vi "TagDB Write Data Example.vi"() -> ()   [LabVIEW 2017]
uses:
  TagDB Application Example/DEF-SineSettings.ctl
  9d9cadb0-fa1b-4c2f-b358-df9a280cddfa.vi
  ba25bb52-5bf6-43af-959d-e9a790955eeb.vi
  c988338c-dfcd-45ae-a170-0c12240f6647.vi
  TagDB/_Support/DataAccess/data-Write.vi
  TagDB/_Support/Error/_[error50000]Invalid DB REF.vi
  TagDB/_Support/DataAccess/TagDB Ref to DVR.vi
  TagDB/_Support/DataAccess/_NameCacher.vi
  TagDB/_Support/DataAccess/_datatypeChecker.vi
  <vilib>/Utility/Data Type/Get Type Information.vi
  TagDB/_Support/Error/_Build Error Cluster.vi
  TagDB/TagDB.lvlib
panel:
  out "Write Tag":string[](array[string])
  out "Write Data Recursive":string[](array[string])
  out "Write Data Elements":string[](array[string])
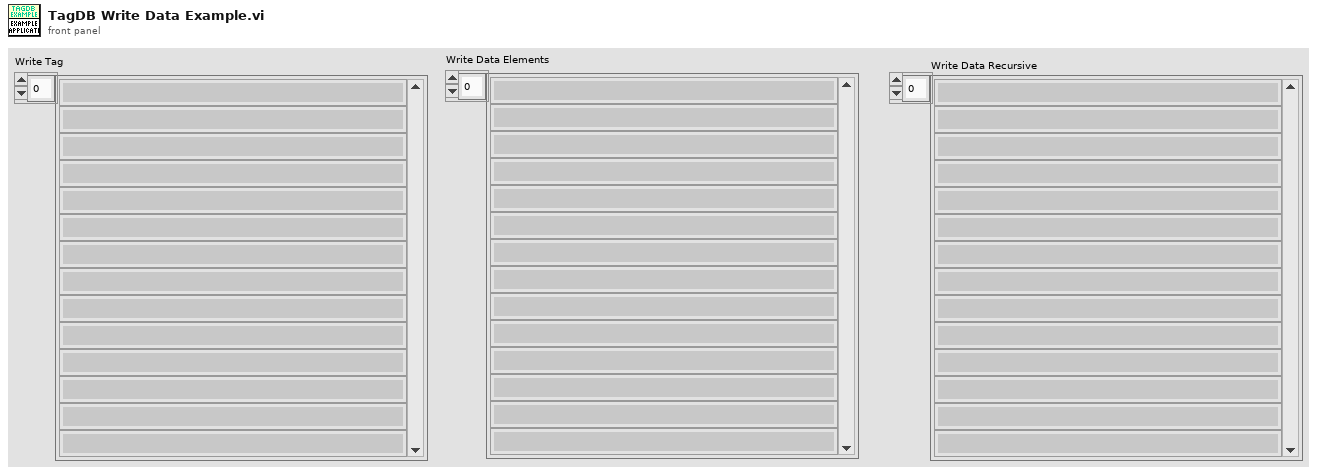
[diagram p1: front panel]
types:
  T1 = typedef "DEF-SineSettings.ctl" = cluster{"frequency":dbl, "amplitude":dbl, "phase":dbl, "sampling info":cluster{"Fs":dbl, "#s":dbl}}
  T2 = typedef "TagDB.lvlib/TagDB.ctl" = refnum<k1>
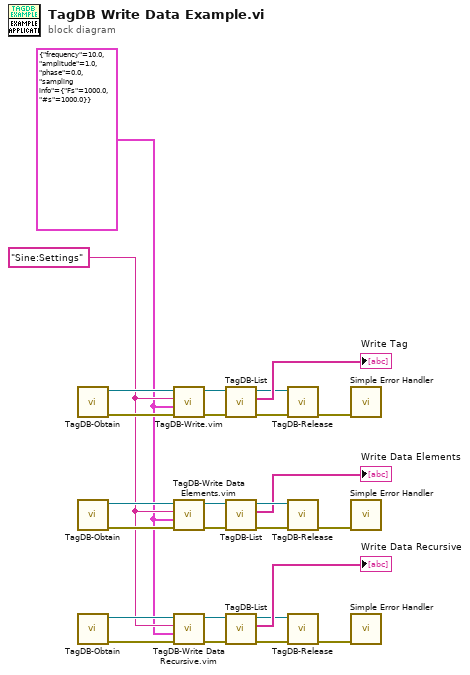
[diagram p0: block diagram]
diagram:
  w2 = "Sine:Settings" ("name")
  w1 = T1 {"frequency"=10.0, "amplitude"=1.0, "phase"=0.0, "sampling info"={"Fs"=1000.0, "#s"=1000.0}} ("Sine Settings")
  n1 = call "TagDB-Obtain.vi"() -> ("error out"=w5:errorcluster, "TagDB"=w4:T2)  [unwired: 5 in, 1 out]
  n2 = call "TagDB-Obtain.vi"() -> ("error out"=w24:errorcluster, "TagDB"=w25:T2)  [unwired: 5 in, 1 out]
  n3 = call "TagDB-Obtain.vi"() -> ("error out"=w13:errorcluster, "TagDB"=w12:T2)  [unwired: 5 in, 1 out]
  n4 = call "TagDB-Write.vim"("error in (no error)"=w5, "Value"=w1, "tag"=w2, "TagDB"=w4) -> ("error out"=w8:errorcluster, "TagDB(dup)"=w6:T2)  [unwired: 5 in, 1 out]
  n5 = call "TagDB-Write Data Elements.vim"("error in (no error)"=w24, "Value"=w1, "root tag"=w2, "TagDB"=w25) -> ("error out"=w21:errorcluster, "TagDB(dup)"=w23:T2)  [unwired: 5 in, 1 out]
  n6 = call "TagDB-Write Data Recursive.vim"("error in (no error)"=w13, "Value"=w1, "root tag"=w2, "TagDB"=w12) -> ("error out"=w16:errorcluster, "TagDB(dup)"=w14:T2)  [unwired: 5 in, 1 out]
  n7 = call "TagDB-List.vi"("error in (no error)"=w8, "TagDB"=w6) -> ("error out"=w9:errorcluster, "names"=→"Write Tag":string[], "TagDB(dup)"=w7:T2)  [unwired: 6 in, 1 out]
  n8 = call "TagDB-List.vi"("error in (no error)"=w21, "TagDB"=w23) -> ("error out"=w20:errorcluster, "names"=→"Write Data Elements":string[], "TagDB(dup)"=w22:T2)  [unwired: 6 in, 1 out]
  n9 = call "TagDB-List.vi"("error in (no error)"=w16, "TagDB"=w14) -> ("error out"=w17:errorcluster, "names"=→"Write Data Recursive":string[], "TagDB(dup)"=w15:T2)  [unwired: 6 in, 1 out]
  n10 = call "TagDB-Release.vi"("error in (no error)"=w9, "TagDB"=w7) -> ("error out"=w3:errorcluster)  [unwired: 9 in]
  n11 = call "TagDB-Release.vi"("error in (no error)"=w20, "TagDB"=w22) -> ("error out"=w26:errorcluster)  [unwired: 9 in]
  n12 = call "TagDB-Release.vi"("error in (no error)"=w17, "TagDB"=w15) -> ("error out"=w11:errorcluster)  [unwired: 9 in]
  n13 = call <vilib>:"Simple Error Handler.vi"("error in (no error)"=w3) -> ()  [unwired: 4 in, 5 out]
  n14 = call <vilib>:"Simple Error Handler.vi"("error in (no error)"=w26) -> ()  [unwired: 4 in, 5 out]
  n15 = call <vilib>:"Simple Error Handler.vi"("error in (no error)"=w11) -> ()  [unwired: 4 in, 5 out]
